vi "OLDLogging Bin Message Loop.vi"(8 "error in (no error)":errorcluster, 10 "Data Queue":refnum<queue>, 11 "Message Queues":T1) -> (0 "error out":errorcluster)   [LabVIEW 2017, in "Logging.lvlib"]
uses:
  Logging.lvlib
  support/Message Queue/All Message Queues.ctl
  support/Message Queue/Message Cluster.ctl
  Logging Configuration.ctl
  Logging State.ctl
  support/Message Queue/Enqueue Message (Single).vi
  <vilib>/Utility/error.llb/Error Cluster From Error Code.vi
  <vilib>/ErrorRing/Error Ring.xnode
  support/Message Queue/Message Queue.lvlib
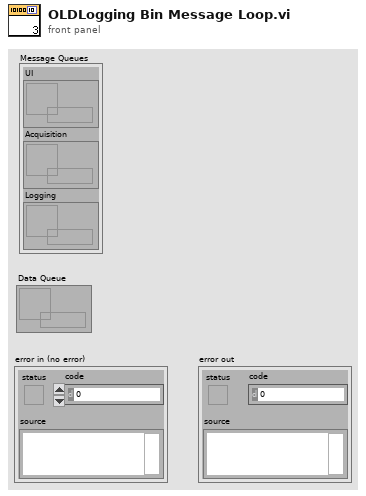
[diagram p1: front panel]
types:
  T1 = typedef "Message Queue.lvlib/All Message Queues.ctl" = cluster{"UI":refnum<queue>, "Acquisition":refnum<queue>, "Logging":refnum<queue>}
  T2 = typedef "Logging.lvlib/Logging Configuration.ctl" = cluster{"Log File Base Path":path, "TDMS File Reference":refnum<k34>, "Log File Offsite Path":path, "Offsite storage?":bool, "Project code":string, "Max writing time to a file [min]":dbl, "refnum out":refnum<file>}
  T3 = enum16{"open", "replace", "create", "open or create", "replace or create", "replace or create with confirmation"}
  T4 = typedef "Logging.lvlib/Logging State.ctl" = enum16{"Idle", "Logging"}
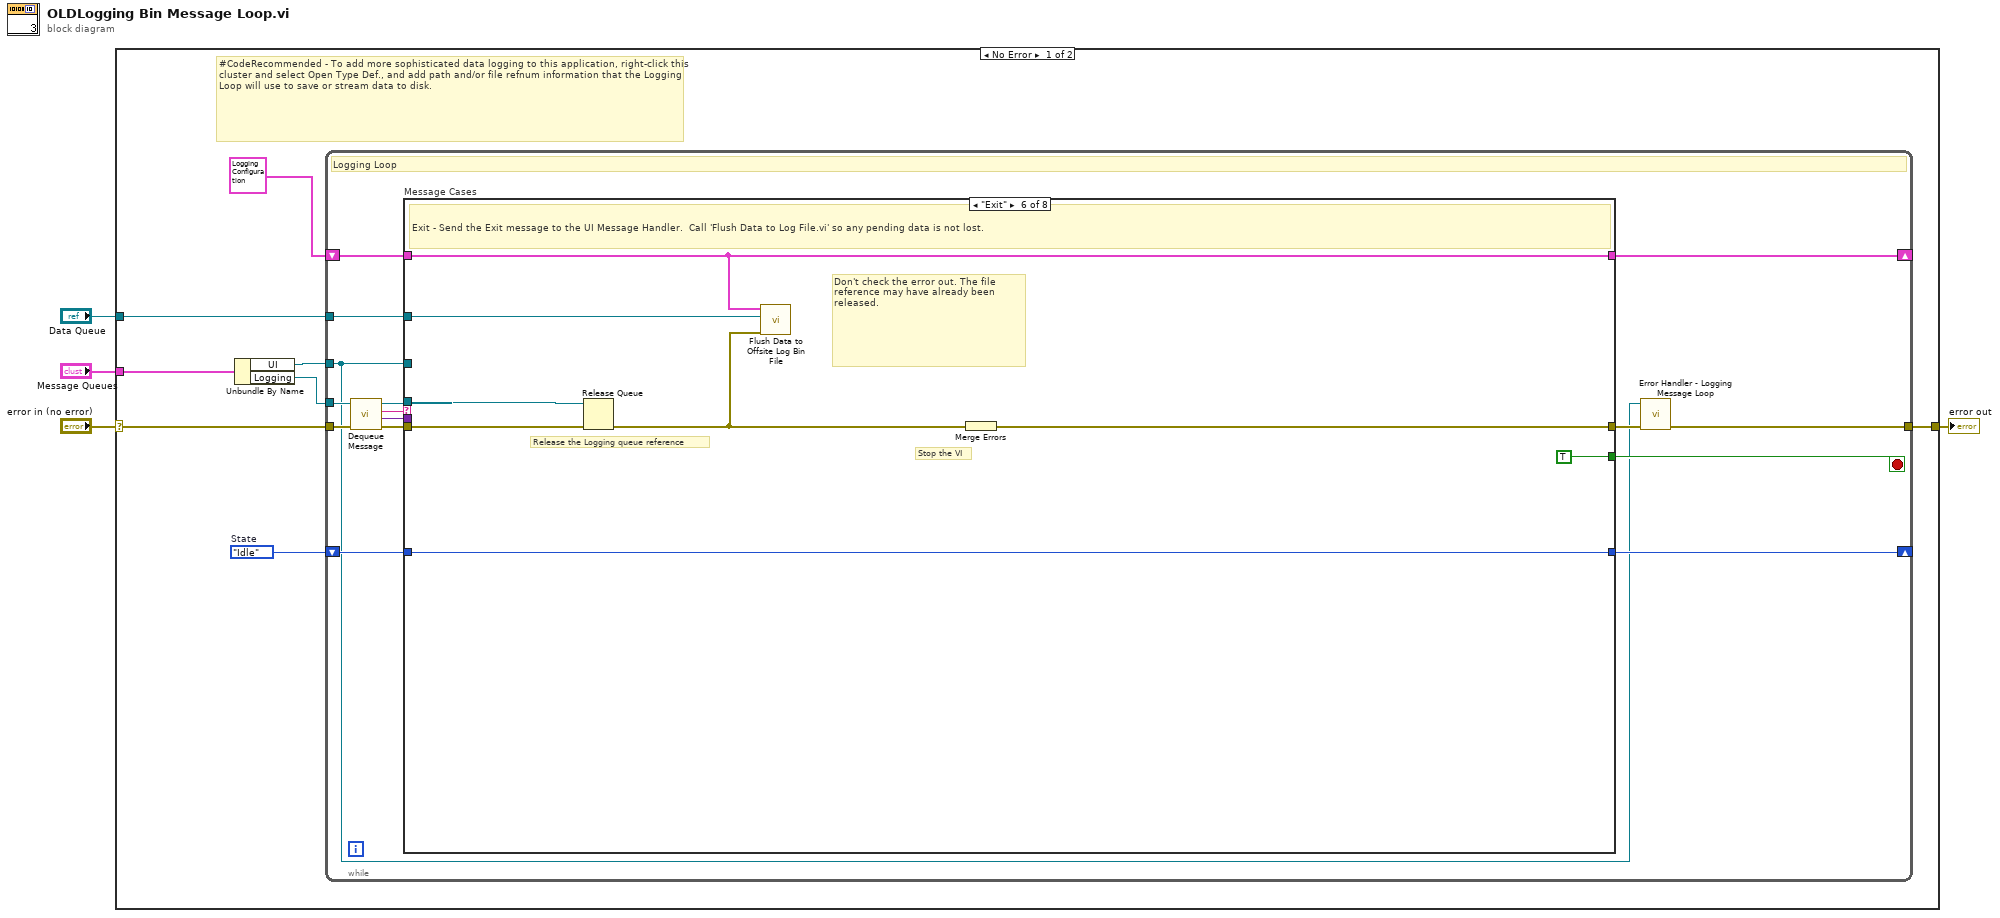
[diagram p0: block diagram]
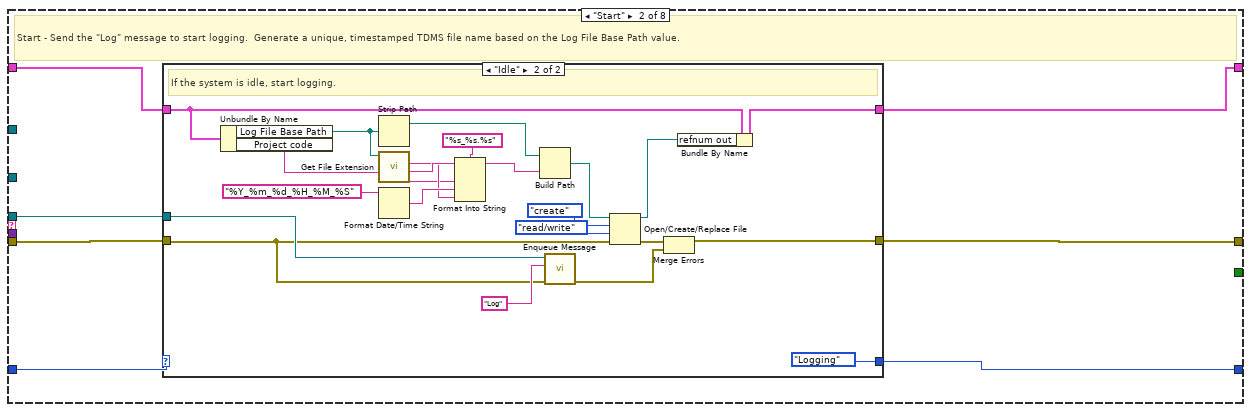
[diagram p3: hidden frame]
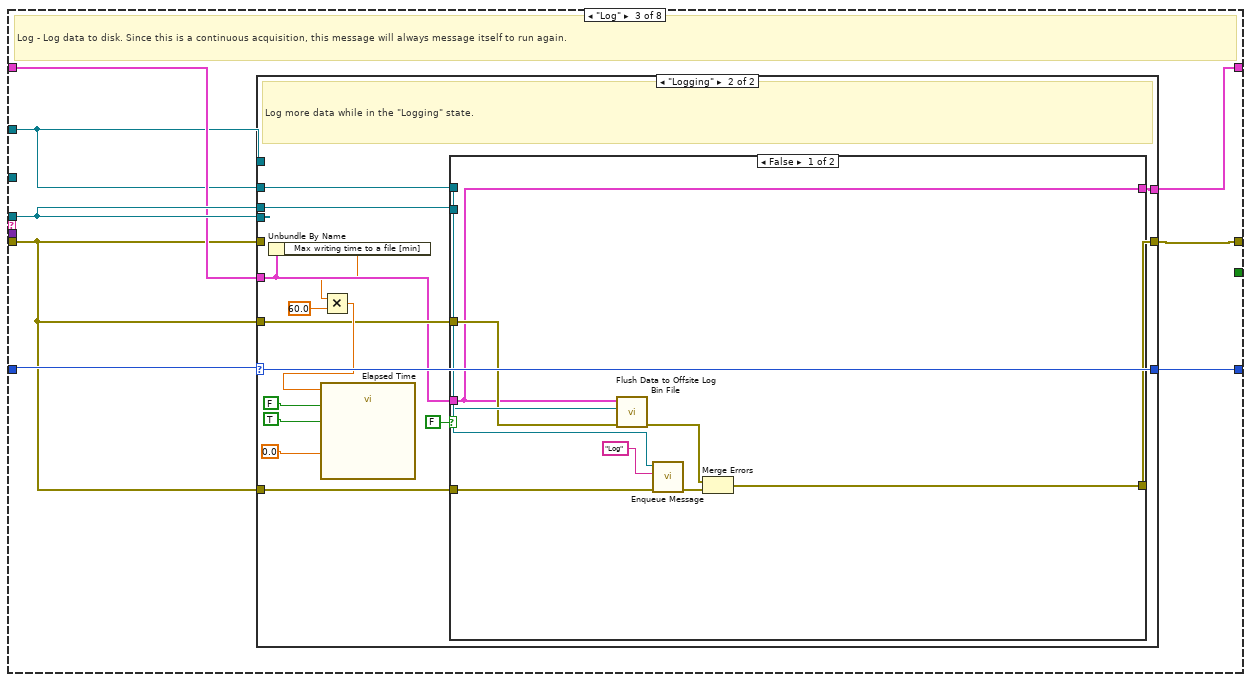
[diagram p5: hidden frame]
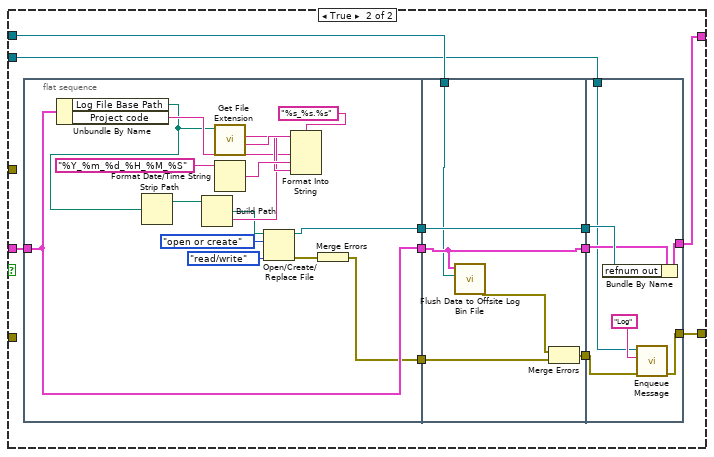
[diagram p7: hidden frame]
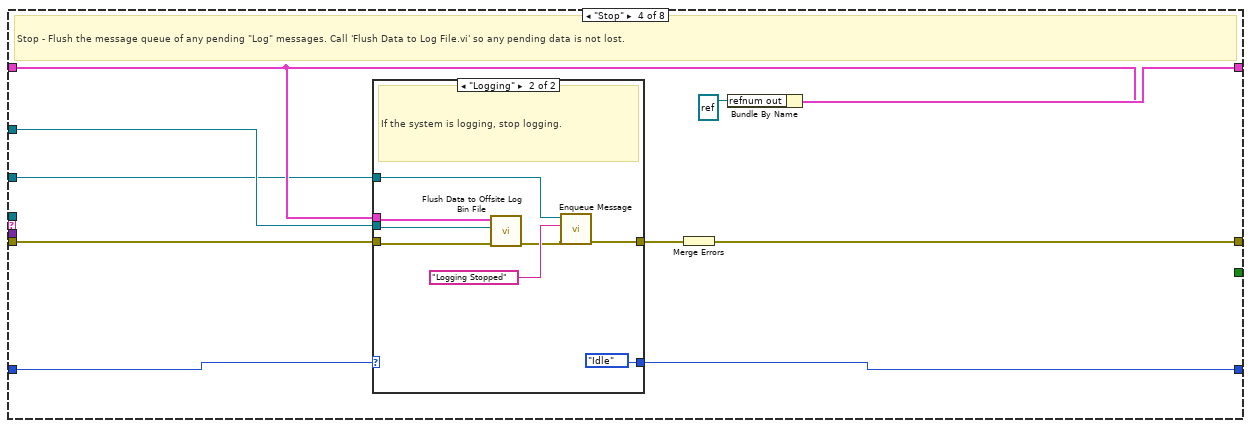
[diagram p8: hidden frame]
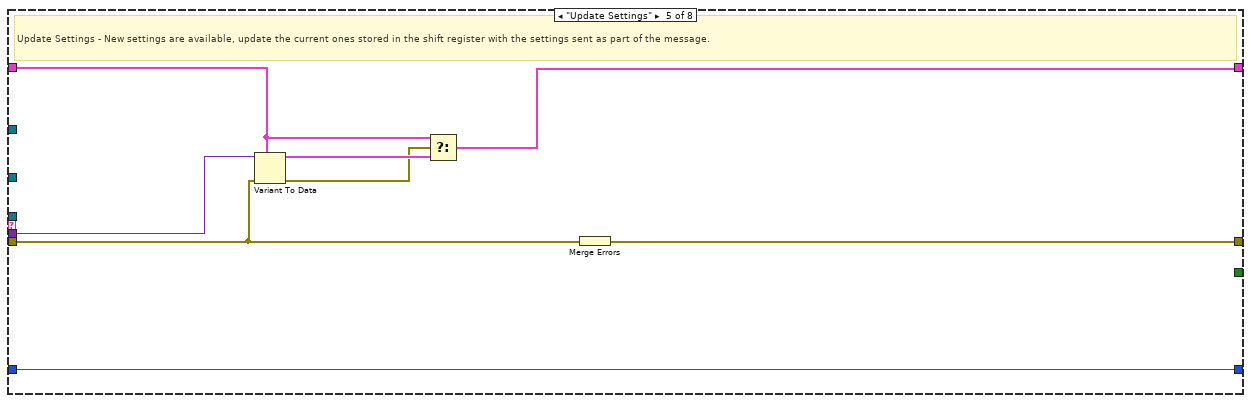
[diagram p10: hidden frame]
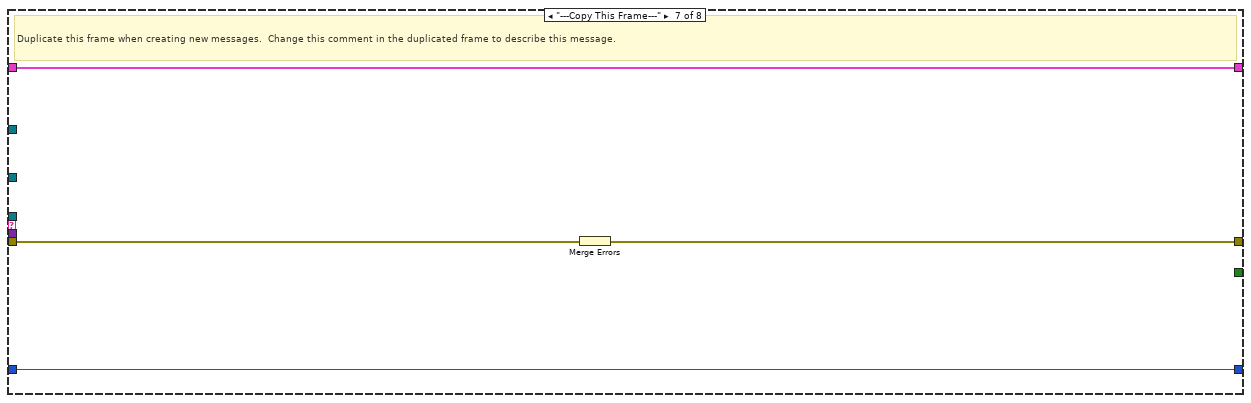
[diagram p11: hidden frame]
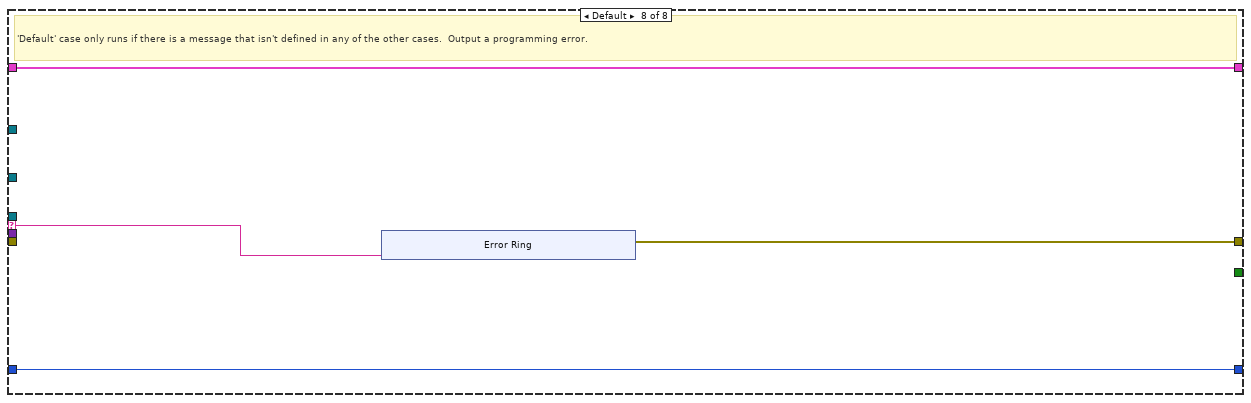
[diagram p12: hidden frame]
diagram:
  n1 = case shown="No Error" "error in (no error)" {
    selector: "error in (no error)" -> [w8 w189]
    tunnel: "Message Queues" -> [w12 _]
    tunnel: [w10 w189] -> w3
    tunnel: "Data Queue" -> [w7 _]
    frame No Error {
      w5 = Logging_State."Idle"  # State
      # "#CodeRecommended - To add more sophisticated data logging to this application, right-click this cluster and select Open Type Def., and add path and/or file refnum information that the Logging Loop will use to save or stream data to disk."
      n2 = Unbundle By Name(w12) -> ("UI"=w6:refnum<queue>, "Logging"=w11:refnum<queue>)
      n3 = while {
        tunnel: w11 -> [w21]
        shift-right: [w27] -> _
        shift-left: T2 {"Log File Base Path"=path "", "TDMS File Reference"=refnum, "Log File Offsite Path"=path "", "Offsite storage?"=FALSE, "Project code"="", "Max writing time to a file [min]"=0.0, "refnum out"=refnum} ("Logging Configuration") -> [w14]
        tunnel: w6 -> [w15]
        tunnel: w7 -> [w20]
        shift-right: [w18] -> _
        shift-left: w5 -> [w19]
        tunnel: w8 -> [w25]
        tunnel: [w17] -> w10
        stop <- w26 stop-if-true
        # "Logging Loop"
        n4 = call "Dequeue Message.vi"("error in (no error)"=w25, "Message Queue"=w21) -> ("error out"=w24:errorcluster, "Message Data"=w23:variant, "Message"=w13:string, "dup Message Queue"=w22:refnum<queue>)  [unwired: 6 in]
        n5 = case "Message Cases" shown="\"Exit\"" w13 {
          selector: w13 -> [_ _ _ _ _ _ _ w178]
          tunnel: w22 -> [_ w36 w68 _ _ w170 _ _]
          tunnel: w24 -> [w29 w35 w65 w142 w159 w171 w177 _]
          tunnel: [w29 w37 w63 w147 w165 w172 w175 w179] -> w16
          tunnel: w14 -> [w30 w32 w67 w143 w163 w168 w176 w181]
          tunnel: [w30 w34 w64 w145 w160 w168 w176 w181] -> w27
          tunnel: [_ _ _ _ _ TRUE _ _] -> w26
          tunnel: w23 -> [_ _ _ _ w164 _ _ _]
          tunnel: w15 -> [_ _ _ w139 _ _ _ _]
          tunnel: w20 -> [_ _ w66 w144 _ w167 _ _]
          tunnel: w19 -> [w28 w31 w70 w141 w158 w169 w174 w180]
          tunnel: [w28 w33 w69 w140 w158 w169 w174 w180] -> w18
          frame "Initialize" {
            # "Initialize - gets called when first launched. Currently a no-op."
          }
          frame "Start" {
            # "Start - Send the \"Log\" message to start logging.  Generate a unique, timestamped TDMS file name based on the Log File Base Path value."
            n6 = case shown="\"Idle\"" w31 {
              selector: w31 -> [w39 _]
              tunnel: [w38 w46] -> w37
              tunnel: w36 -> [_ w47]
              tunnel: w35 -> [w38 w45]
              tunnel: w32 -> [w40 w41]
              tunnel: [w40 w49] -> w34
              tunnel: [w39 Logging_State."Logging" ("State")] -> w33
              frame "Logging" {
                # "The system is already logging. Ignore the \"Start\" message."
              }
              frame "Idle" {
                # "If the system is idle, start logging."
                n7 = Unbundle By Name(w41) -> ("Log File Base Path"=w61:path, "Project code"=w44:string)
                n8 = Strip Path(path=w61) -> (stripped path=w58:path)  [unwired: 1 out]
                n9 = call <vilib>:"Get File Extension.vi"("file"=w61) -> ("filename without extension"=w59:string, "lowercase file extension"=w55:string)  [unwired: 6 in, 3 out]
                n10 = Format Date/Time String(time format string (%c)="%Y_%m_%d_%H_%M_%S") -> (date/time string=w56:string)  [unwired: 2 in]
                n11 = Format Into String(format string="%s_%s.%s", initial string=w59, w44, w56, w55) -> (resulting string=w54:string)  [unwired: 1 in, 1 out]
                n12 = Build Path(base path=w58, name or relative path=w54) -> (appended path=w53:path)
                n13 = call-poly "Enqueue Message.vi"("error in (no error)"=w45, "Message"="Log", "Message Queue"=w47) -> ("error out"=w51:errorcluster)  [unwired: 7 in, 1 out]
                n14 = Open/Create/Replace File(file path (use dialog)=w53, error in=w45, operation (0:open)=T3."create", access (0:read/write)=enum16{"read/write", "read-only", "write-only"}."read/write") -> (refnum out=w42:refnum<file>, error out=w52:errorcluster)  [unwired: 2 in, 1 out]
                n15 = Merge Errors(w52, w51) -> (w46:errorcluster)
                n16 = Bundle By Name(cluster=w41, "refnum out"=w42) -> (w49:T2)
              }
            }
          }
          frame "Log" {
            # "Log - Log data to disk. Since this is a continuous acquisition, this message will always message itself to run again."
            n17 = case shown="\"Logging\"" w70 {
              selector: w70 -> [w73 w87]
              tunnel: [w72 w75] -> w63
              tunnel: w68 -> [_ _]
              tunnel: w66 -> [_ _]
              tunnel: w65 -> [w72 _]
              tunnel: [w73 w87] -> w69
              tunnel: w65 -> [_ w82]
              tunnel: w68 -> [_ w81]
              tunnel: w67 -> [w71 w78]
              tunnel: w66 -> [_ w80]
              tunnel: w65 -> [_ w79]
              tunnel: [w71 w76] -> w64
              frame "Idle" {
                # "Ignore \"Log\" messages when the logging is idle."
              }
              frame "Logging" {
                # "Log more data while in the \"Logging\" state."
                n18 = Unbundle By Name(w78) -> ("Max writing time to a file [min]"=w77:dbl)
                n19 = Multiply(x=w77, y=60.0) -> (x*y=w86:dbl)
                n20 = call "Elapsed Time"("Time Target (s)"=w86, "Reset"=FALSE, "Auto Reset"=TRUE, "Set Start Time (s)"=0.0) -> ()  [unwired: 8 in, 8 out]
                n21 = case shown="False" FALSE {
                  tunnel: w82 -> [w96 _]
                  tunnel: w81 -> [w94 w98]
                  tunnel: w78 -> [w90 w106]
                  tunnel: w80 -> [w93 w102]
                  tunnel: w79 -> [w92 _]
                  tunnel: [w91 w99] -> w75
                  tunnel: [w90 w105] -> w76
                  frame False {
                    n22 = call "Flush Data to Offsite Log Bin File.vi"("Logging Configuration"=w90, "Data Queue"=w93, "error in (no error)"=w92) -> ("error out"=w97:errorcluster)  [unwired: 7 in]
                    n23 = call-poly "Enqueue Message.vi"("error in (no error)"=w96, "Message"="Log", "Message Queue"=w94) -> ("error out"=w89:errorcluster)  [unwired: 7 in, 1 out]
                    n24 = Merge Errors(w97, w89) -> (w91:errorcluster)
                  }
                  frame True {
                    n25 = flat-sequence {
                      tunnel: [w112] -> w107
                      tunnel: w106 -> [w112]
                      tunnel: [w111] -> w103
                      tunnel: [w110] -> w101
                      tunnel: [w128] -> w108
                      tunnel: w107 -> [w128]
                      tunnel: [w129] -> w104
                      tunnel: w103 -> [w129]
                      tunnel: w102 -> [w127]
                      tunnel: w101 -> [w126]
                      tunnel: [w125] -> w100
                      tunnel: [w135] -> w105
                      tunnel: w108 -> [w136]
                      tunnel: w104 -> [w137]
                      tunnel: w100 -> [w133]
                      tunnel: [w132] -> w99
                      tunnel: w98 -> [w131]
                      frame #0 {
                        n26 = Unbundle By Name(w112) -> ("Log File Base Path"=w109:path, "Project code"=w113:string)
                        n27 = Strip Path(path=w109) -> (stripped path=w123:path)  [unwired: 1 out]
                        n28 = call <vilib>:"Get File Extension.vi"("file"=w109) -> ("filename without extension"=w124:string, "lowercase file extension"=w121:string)  [unwired: 6 in, 3 out]
                        n29 = Format Date/Time String(time format string (%c)="%Y_%m_%d_%H_%M_%S") -> (date/time string=w122:string)  [unwired: 2 in]
                        n30 = Format Into String(format string="%s_%s.%s", initial string=w124, w113, w122, w121) -> (resulting string=w120:string)  [unwired: 1 in, 1 out]
                        n31 = Build Path(base path=w123, name or relative path=w120) -> (appended path=w119:path)
                        n32 = Open/Create/Replace File(file path (use dialog)=w119, operation (0:open)=T3."open or create", access (0:read/write)=enum16{"read/write", "read-only", "write-only"}."read/write") -> (refnum out=w111:refnum<file>, error out=w118:errorcluster)  [unwired: 3 in, 1 out]
                        n33 = Merge Errors(w118) -> (w110:errorcluster)
                      }
                      frame #1 {
                        n34 = call "Flush Data to Offsite Log Bin File.vi"("Logging Configuration"=w128, "Data Queue"=w127) -> ("error out"=w130:errorcluster)  [unwired: 8 in]
                        n35 = Merge Errors(w130, w126) -> (w125:errorcluster)
                      }
                      frame #2 {
                        n36 = Bundle By Name(cluster=w136, "refnum out"=w137) -> (w135:T2)
                        n37 = call-poly "Enqueue Message.vi"("error in (no error)"=w133, "Message"="Log", "Message Queue"=w131) -> ("error out"=w132:errorcluster)  [unwired: 7 in, 1 out]
                      }
                    }
                  }
                }
              }
            }
          }
          frame "Stop" {
            # "Stop - Flush the message queue of any pending \"Log\" messages. Call 'Flush Data to Log File.vi' so any pending data is not lost."
            n38 = case shown="\"Logging\"" w141 {
              selector: w141 -> [w148 _]
              tunnel: [w149 w156] -> w146
              tunnel: w144 -> [_ w152]
              tunnel: w143 -> [_ w153]
              tunnel: w142 -> [w149 w151]
              tunnel: [w148 Logging_State."Idle" ("State")] -> w140
              tunnel: w139 -> [_ w155]
              frame "Idle" {
                # "The system is already idle. Ignore the \"Stop\" message."
              }
              frame "Logging" {
                # "If the system is logging, stop logging."
                n39 = call "Flush Data to Offsite Log Bin File.vi"("Logging Configuration"=w153, "Data Queue"=w152, "error in (no error)"=w151) -> ("error out"=w150:errorcluster)  [unwired: 7 in]
                n40 = call-poly "Enqueue Message.vi"("error in (no error)"=w150, "Message"="Logging Stopped", "Message Queue"=w155) -> ("error out"=w156:errorcluster)  [unwired: 7 in, 1 out]
              }
            }
            n41 = Merge Errors(w146) -> (w147:errorcluster)
            n42 = Bundle By Name(cluster=w143, "refnum out"=refnum<file> refnum) -> (w145:T2)
          }
          frame "Update Settings" {
            # "Update Settings - New settings are available, update the current ones stored in the shift register with the settings sent as part of the message."
            n43 = Variant To Data(error in=w159, type=w163, Variant=w164) -> (data=w162:T2, error out=w161:errorcluster)
            n44 = Select(t=w163, s=w161, f=w162) -> (s? t:f=w160:T2)
            n45 = Merge Errors(w159) -> (w165:errorcluster)
          }
          frame "Exit" {
            # "Don't check the error out. The file reference may have already been released."
            # "Release the Logging queue reference"
            # "Stop the VI"
            # "Exit - Send the Exit message to the UI Message Handler.  Call 'Flush Data to Log File.vi' so any pending data is not lost."
            n46 = Release Queue(queue=w170, error in (no error)=w171) -> (error out=w166:errorcluster)  [unwired: 1 in, 2 out]
            n47 = call "Flush Data to Offsite Log Bin File.vi"("Logging Configuration"=w168, "Data Queue"=w167, "error in (no error)"=w166) -> ()  [unwired: 7 in, 1 out]
            n48 = Merge Errors(w166) -> (w172:errorcluster)
          }
          frame "---Copy This Frame---" {
            # "Duplicate this frame when creating new messages.  Change this comment in the duplicated frame to describe this message."
            n49 = Merge Errors(w177) -> (w175:errorcluster)
          }
          frame Default {
            # "'Default' case only runs if there is a message that isn't defined in any of the other cases.  Output a programming error."
            n50 = xnode "Error Ring"("parameter 0"=w178) -> ("error out"=w179:errorcluster)
          }
        }
        n51 = call "Error Handler - Logging Message Loop.vi"("error in (no error)"=w16, "Message Queue"=w15) -> ("dup error in"=w17:errorcluster)  [unwired: 8 in, 1 out]
      }
    }
    frame Error {
    }
  }
  "error out" <- w3
